vi "Detect (sub vi).vi"(8 "MOVE position":i32[](array[numeric]), 9 "Points position":i32[][](array[numeric]), 10 "Display":u32[][](array[colorbox]), 11 "Points":i32) -> (1 "Points 2":i32, 2 "Display 2":u32[][](array[colorbox]), 3 "Points position 2":i32[][](array[numeric]))   [LabVIEW 2014]
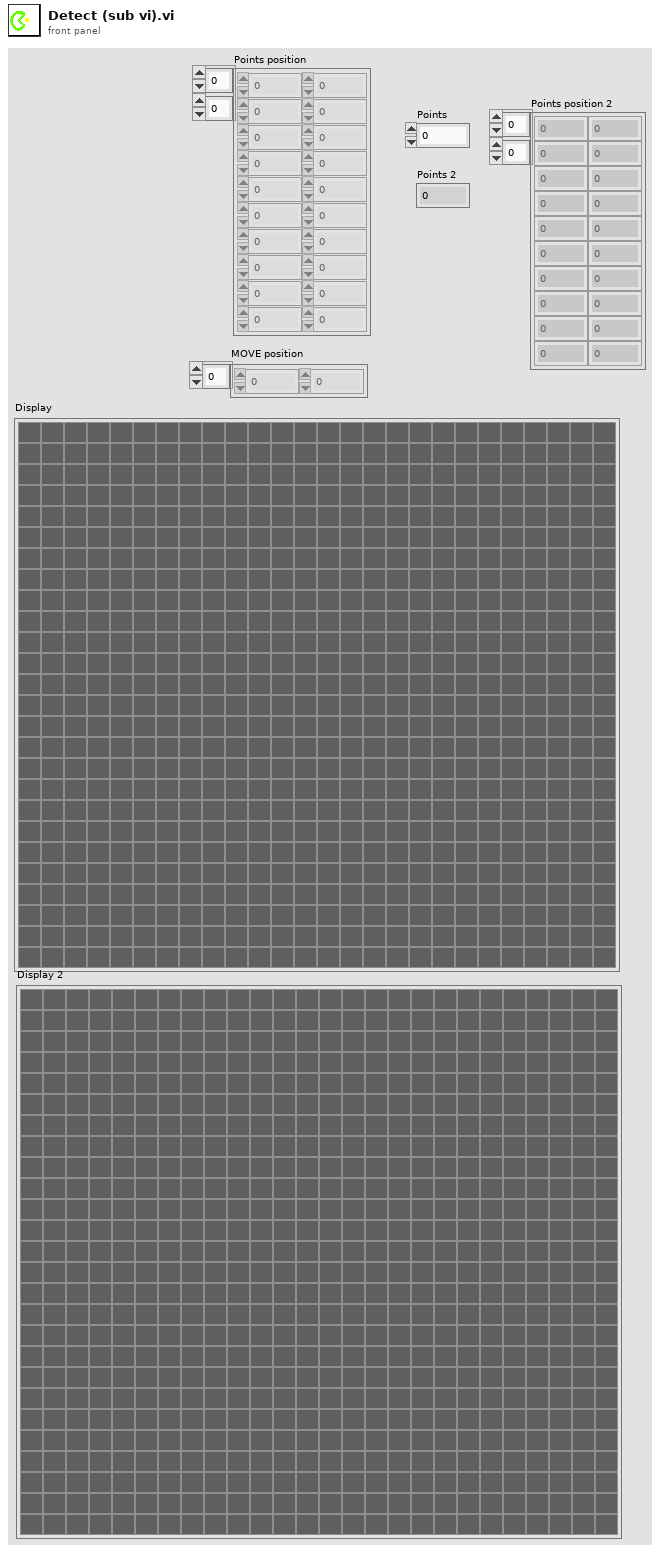
[diagram p1: front panel]
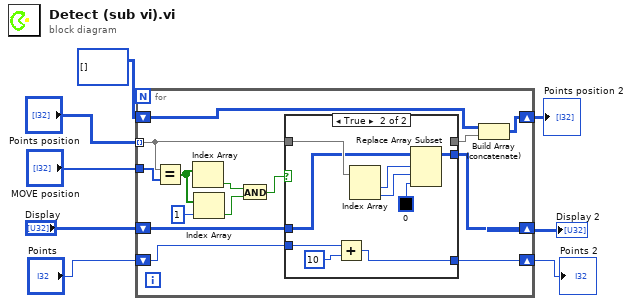
[diagram p0: block diagram]
diagram:
  n1 = for {
    tunnel: "Points position" -> [w16] mode=indexing
    tunnel: "MOVE position" -> [w22]
    shift-right: [w14] -> w5
    shift-left: "Display" -> [w15]
    shift-right: [w12] -> w3
    shift-left: "Points" -> [w13]
    shift-right: [w10] -> w1
    shift-left: i32[][] [] -> [w9]
    n2 = Equal?(x=w16, y=w22) -> (x = y?=w21:bool[])
    n3 = Index Array(array=w21) -> (element=w18:bool)  [unwired: 1 in]
    n4 = Index Array(array=w21, index=1) -> (element=w19:bool)
    n5 = And(x=w18, y=w19) -> (x .and. y?=w17:bool)
    n6 = case shown="True" w17 {
      tunnel: w16 -> [w23 w31]
      tunnel: w15 -> [w25 w30]
      tunnel: [w25 w29] -> w14
      tunnel: w13 -> [w24 w28]
      tunnel: [w24 w27] -> w12
      tunnel: [w23 _] -> w11
      frame False {
      }
      frame True {
        n7 = Add(x=w28, y=10) -> (x+y=w27:i32)
        n8 = Index Array(array=w31) -> (element #1=w32:i32, element #2=w33:i32)  [unwired: 2 in]
        n9 = Replace Array Subset(array=w30, new element=u32 0 ("Color Box"), index (row)=w32, index (col)=w33) -> (w29:u32[][])
      }
    }
    n10 = Build Array (concatenate)(w9, w11) -> (w10:i32[][])
  }
  "Display 2" <- w5
  "Points 2" <- w3
  "Points position 2" <- w1
